vi "SendRelayProtocol.vi"(7 "Send":bool, 9 "Initialize":bool, 10 "Relay prev":T1={"type"="Relay", "device"="", "name"="", "data"={"<init_fwd"=FALSE, "<init_rev"=FALSE, "<fwd"=FALSE, "<rev"=FALSE}}, 11 "Relay new":T1={"type"="Relay", "device"="", "name"="", "data"={"<init_fwd"=FALSE, "<init_rev"=FALSE, "<fwd"=FALSE, "<rev"=FALSE}}) -> ()   [LabVIEW 2019]
uses:
  Relay proto.ctl
  Relay data proto.ctl
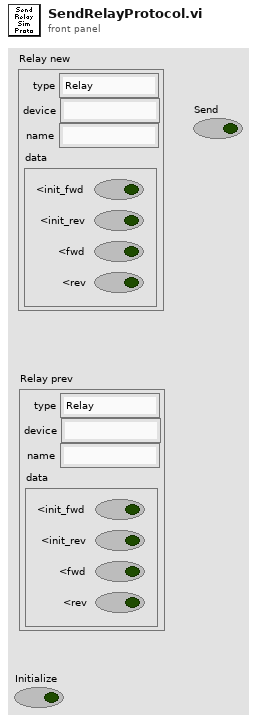
[diagram p1: front panel]
types:
  T1 = typedef "Relay proto.ctl" = cluster{"type":string, "device":string, "name":string, "data":T2}
  T2 = typedef "Relay data proto.ctl" = cluster{"<init_fwd":bool, "<init_rev":bool, "<fwd":bool, "<rev":bool}
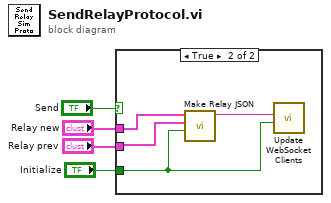
[diagram p0: block diagram]
diagram:
  n1 = case shown="True" "Send" {
    tunnel: "Relay new" -> [_ w6]
    tunnel: "Relay prev" -> [_ w5]
    tunnel: "Initialize" -> [_ w8]
    frame False {
    }
    frame True {
      n2 = call "Make Relay JSON.vi"("Force"=w8, "Relay prev"=w5, "Relay new"=w6) -> ("delta JSON"=w7:string)  [unwired: 8 in]
      n3 = call "Update WebSocket Clients.vi"("Initialize"=w8, "delta JSON"=w7) -> ()  [unwired: 10 in]
    }
  }
